vi "HEIDOLPH_CONTROL07.vi"(8 "shutdown":bool, 10 "Set RPM":dbl(slide) scale=0.0..500.0, 11 "Device port":dbl=13.0) -> (1 "Dynamic Data":dynamicdata(waveform), 2 "RPM":dbl, 3 "RPM 2":dbl, 4 "Torque":dbl, 5 "Torque 2":dbl)   [LabVIEW 2015]
uses:
  x64/Debug/BERTTA.dll
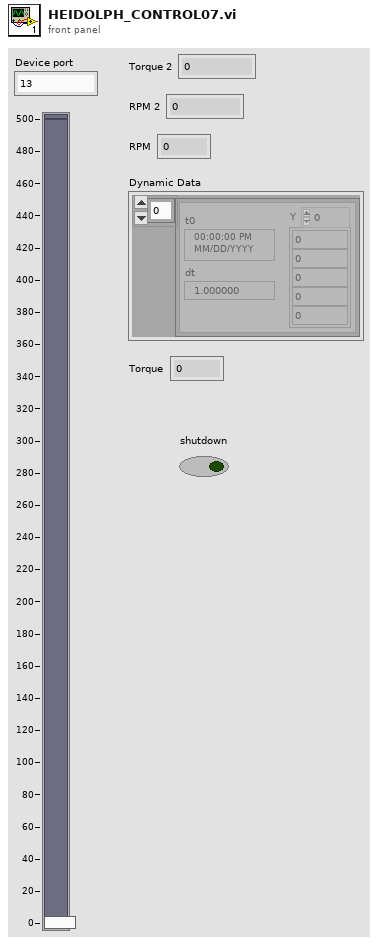
[diagram p1: front panel]
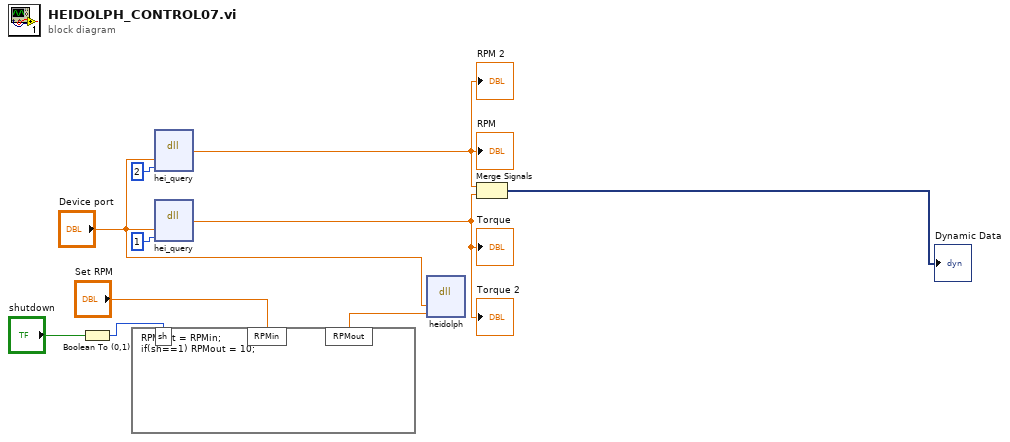
[diagram p0: block diagram]
diagram:
  n1 = Boolean To (0,1)(Boolean="shutdown") -> (0, 1=w3:i16)
  n2 = formula code="RPMout = RPMin;\nif(sh==1) RPMout = 10;"("sh"=w3, "RPMin"="Set RPM") -> ("RPMout"=w1:dbl)
  n3 = dll-call lib="C:/Users/shresplab/OneDrive - Kemira Oyj/Documents/Visual Studio 2017/Projects/Bertta/BERTTA/x64/Debug/BERTTA.dll" fn="hei_query"("port"="Device port", "q"=2) -> ("return type"=w8:dbl)  [unwired: 5 in, 2 out]
  "RPM" <- w8
  "RPM 2" <- w8
  n4 = dll-call lib="C:/Users/shresplab/OneDrive - Kemira Oyj/Documents/Visual Studio 2017/Projects/Bertta/BERTTA/x64/Debug/BERTTA.dll" fn="hei_query"("port"="Device port", "q"=1) -> ("return type"=w9:dbl)  [unwired: 5 in, 2 out]
  "Torque" <- w9
  "Torque 2" <- w9
  n5 = dll-call lib="C:/Users/shresplab/OneDrive - Kemira Oyj/Documents/Visual Studio 2017/Projects/Bertta/BERTTA/x64/Debug/BERTTA.dll" fn="heidolph"("port"="Device port", "speed"=w1) -> ()  [unwired: 6 in, 2 out]
  n6 = Merge Signals(w8, w9) -> (→"Dynamic Data":dynamicdata)
